vi "Read Test Sequence.vi"(11 "Toggle 6 in":refnum<class "Toggle 7.1.lvclass">) -> (2 "Test Sequence":T1, 3 "Toggle 6 out":refnum<class "Toggle 7.1.lvclass">)   [LabVIEW 2020, in "Toggle 7.1.lvclass"]
uses:
  Toggle 7.1.lvclass
  Controls/Test Sequence.ctl
  Controls/Register to Write.ctl
  Controls/EFuse modes enum.ctl
  Toggle 7.1.lvclass/Toggle 7.1.ctl
  PIC-device/PIC-Device.lvclass
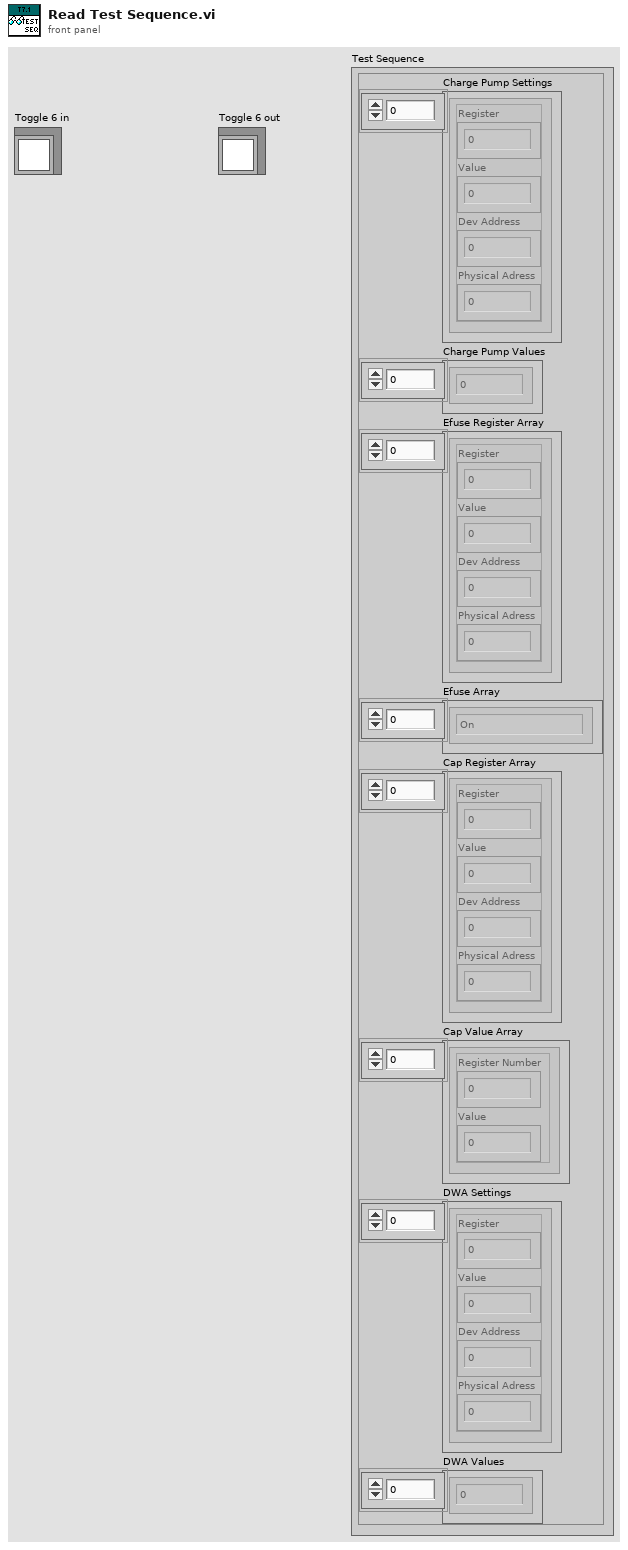
[diagram p1: front panel]
types:
  T1 = typedef "Toggle 7.1.lvclass/Test Sequence.ctl" = cluster{"Charge Pump Settings":T2[], "Charge Pump Values":dbl[], "Efuse Register Array":T2[], "Efuse Array":T3[], "Cap Register Array":T2[], "Cap Value Array":cluster{"Register Number":u32, "Value":dbl}[], "DWA Settings":T2[], "DWA Values":dbl[]}
  T2 = typedef "PIC-Device.lvclass/Register to Write.ctl" = cluster{"Register":u32, "Value":u32, "Dev Address":u32, "Physical Adress":u32}
  T3 = typedef "Toggle 7.1.lvclass/EFuse modes enum.ctl" = enum16{"On", "Off", "Both On and Off"}
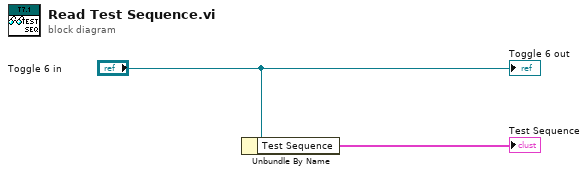
[diagram p0: block diagram]
diagram:
  n1 = Unbundle By Name("Toggle 6 in") -> ("Test Sequence"=→"Test Sequence":T1)
  "Toggle 6 out" <- "Toggle 6 in"
